vi "SetUp Wi-Fi Connection.vi"(8 "error in (no error)":errorcluster, 11 "Wi-Fi Shield in":refnum<class "Wi-Fi Shield.lvclass">) -> (0 "error out":errorcluster, 3 "Wi-Fi Shield out":refnum<class "Wi-Fi Shield.lvclass">)   [LabVIEW 2020, in "Wi-Fi Shield.lvclass"]
uses:
  Wi-Fi Shield.lvclass
  480319c2-f43b-4945-9afd-1c9c5fb20ae1.vi
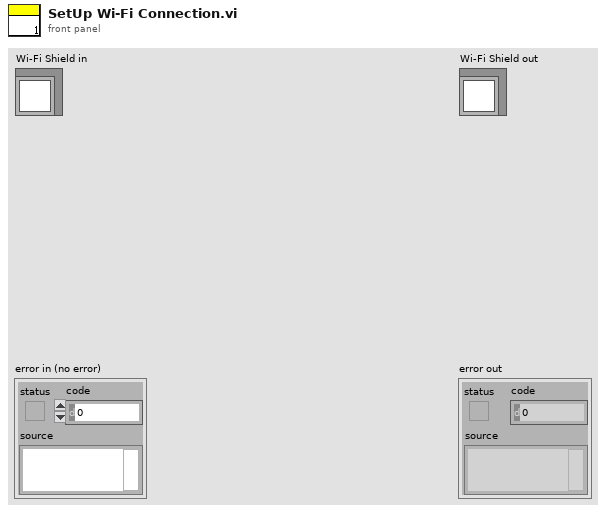
[diagram p1: front panel]
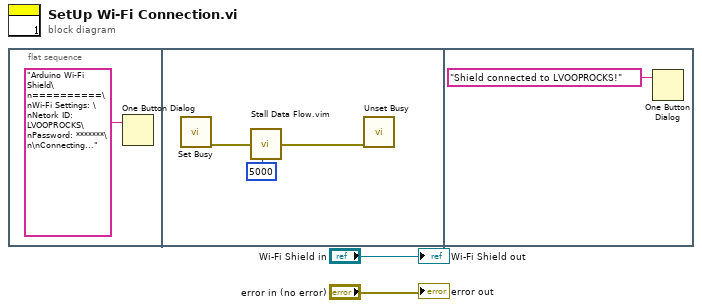
[diagram p0: block diagram]
diagram:
  n1 = flat-sequence {
    frame #0 {
      n2 = One Button Dialog(message="Arduino Wi-Fi Shield\n==========\nWi-Fi Settings: \nNetork ID: LVOOPROCKS\nPassword: *******\n\nConnecting...") -> ()  [unwired: 1 in, 1 out]
    }
    frame #1 {
      n3 = call <vilib>:"Set Busy.vi"() -> ("error out"=w6:errorcluster)  [unwired: 10 in, 1 out]
      n4 = call "Stall Data Flow.vim"("value in"=w6, "milliseconds to wait"=u32 5000) -> ("value out"=w5:errorcluster)  [unwired: 1 out]
      n5 = call <vilib>:"Unset Busy.vi"("error in (no error)"=w5) -> ()  [unwired: 10 in, 1 out]
    }
    frame #2 {
      n6 = One Button Dialog(message="Shield connected to LVOOPROCKS!") -> ()  [unwired: 1 in, 1 out]
    }
  }
  "error out" <- "error in (no error)"
  "Wi-Fi Shield out" <- "Wi-Fi Shield in"
